vi "Create RefNum and Add to Cluster.vi"(8 "error in (no error)":errorcluster, 10 "Owning Cluster in":refnum<vi>, 11 "Controls":refnum<vi>[](array[refnum])) -> (0 "error out":errorcluster, 2 "Owning Cluster out":refnum<vi>, 3 "Created RefNum":refnum<vi>)   [LabVIEW 2020]
uses:
  <vilib>/Utility/miscctls.llb/LVPositionTypeDef.ctl
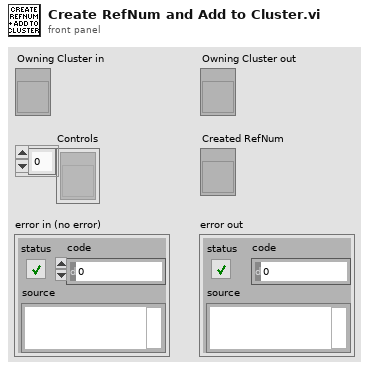
[diagram p1: front panel]
types:
  T1 = typedef "LVPositionTypeDef.ctl" = cluster{"Left":i32, "Top":i32}
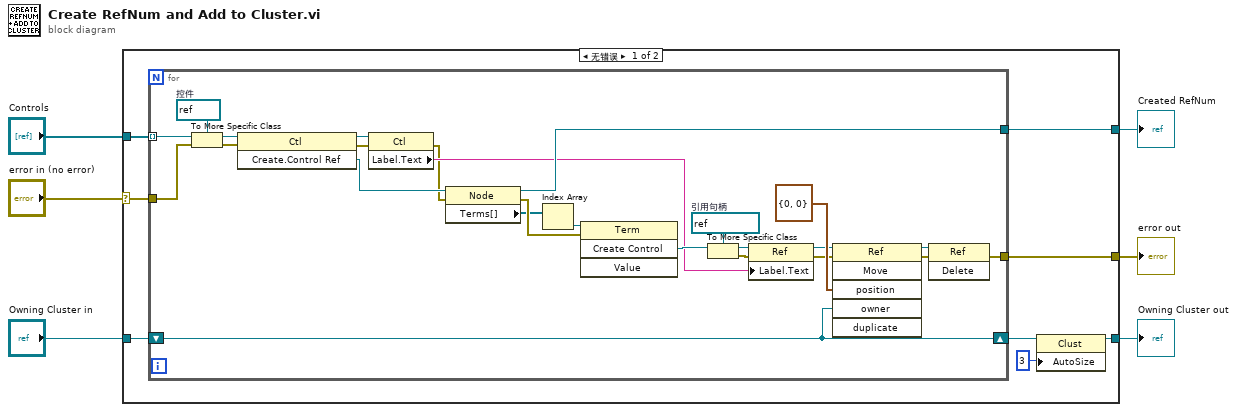
[diagram p0: block diagram]
diagram:
  n1 = case shown="无错误" "error in (no error)" {
    selector: "error in (no error)" -> [w11 w41]
    tunnel: "Owning Cluster in" -> [w14 w40]
    tunnel: [w13 _] -> w5
    tunnel: "Controls" -> [w12 _]
    tunnel: [w7 w40] -> w3
    tunnel: [w10 w41] -> w1
    frame No Error {
      n2 = for {
        tunnel: w12 -> [w27] mode=indexing
        shift-right: [w19] -> w8
        shift-left: w14 -> [w19]
        tunnel: [w34] -> w10
        tunnel: w11 -> [w33]
        tunnel: [w18] -> w13
        w29 = refnum<vi> refnum  # 引用句柄
        w32 = refnum<vi> refnum  # 控件
        n3 = To More Specific Class(target class=w32, reference=w27, error in=w33) -> (specific class reference=w26:refnum<vi>, error out=w39:errorcluster)
        n4 = invoke class="Ctl" method="Create.Control Ref"(reference=w26, error in=w39) -> (reference out=w23:refnum<vi>, error out=w38:errorcluster, "Create Control Ref"=w25:refnum<vi>)  [unwired: 1 in]
        n5 = property class="Ctl"(reference=w23, error in=w38) -> (error out=w16:errorcluster, "Label.Text"=w17:string)  [unwired: 1 out]
        n6 = property class="Node"(reference=w25, error in=w16) -> (reference out=w18:refnum<vi>, error out=w37:errorcluster, "Terms[]"=w31:refnum<vi>[])
        n7 = Index Array(array=w31) -> (element=w30:refnum<vi>)  [unwired: 1 in]
        n8 = invoke class="Term" method="Create Control"(reference=w30, error in=w37) -> ("Create Control"=w24:refnum<vi>)  [unwired: 2 in, 3 out]
        n9 = To More Specific Class(target class=w29, reference=w24) -> (specific class reference=w22:refnum<vi>, error out=w36:errorcluster)  [unwired: 1 in]
        n10 = property class="Ref"(reference=w22, error in=w36, "Label.Text"=w17) -> (reference out=w21:refnum<vi>, error out=w15:errorcluster)
        n11 = invoke class="Ref" method="Move"(reference=w21, error in=w15, "position"=T1 {"Left"=0, "Top"=0}, "owner"=w19) -> (reference out=w20:refnum<vi>, error out=w35:errorcluster)  [unwired: 2 in, 4 out]
        n12 = invoke class="Ref" method="Delete"(reference=w20, error in=w35) -> (error out=w34:errorcluster)  [unwired: 1 in, 2 out]
      }
      n13 = property class="Clust"(reference=w8, "AutoSize"=u32 3 ("Auto Sizing")) -> (reference out=w7:refnum<vi>)  [unwired: 1 in, 1 out]
    }
    frame Error {
    }
  }
  "Created RefNum" <- w5
  "Owning Cluster out" <- w3
  "error out" <- w1
